vi "Init Controls.vi"(8 "error in":errorcluster, 10 "Disabled Controls":string[](array[string]), 11 "VI ref":refnum<vi>) -> (0 "error out":errorcluster)   [LabVIEW 2018]
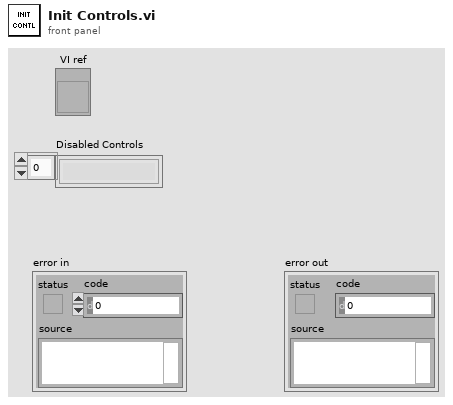
[diagram p1: front panel]
types:
  T1 = enum8{"Enabled", "Disabled", "Disabled and Grayed Out"}
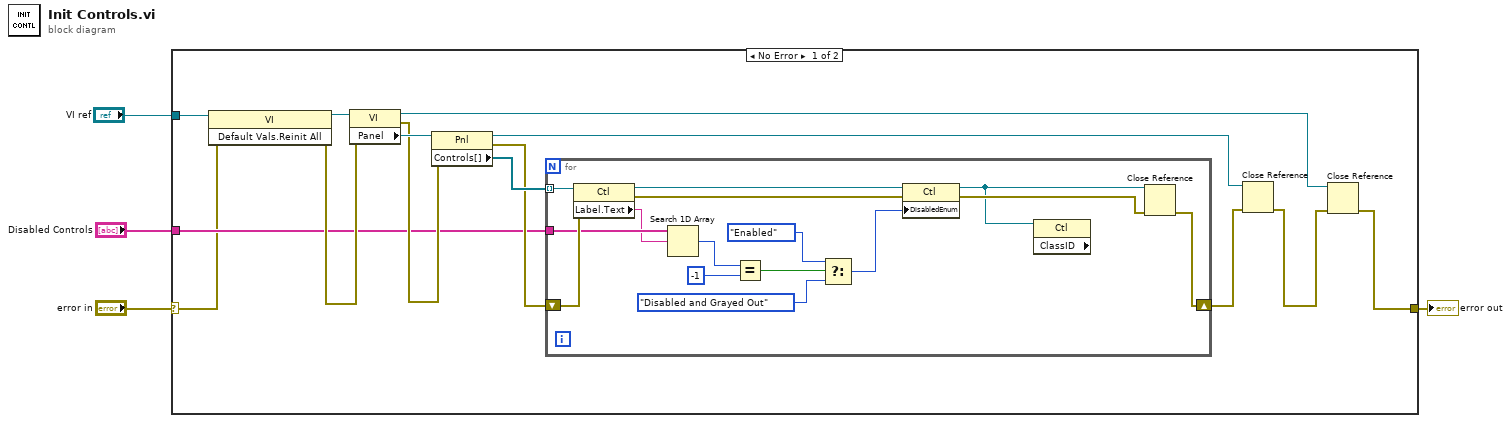
[diagram p0: block diagram]
diagram:
  n1 = case shown="No Error" "error in" {
    selector: "error in" -> [w10 w34]
    tunnel: "VI ref" -> [w18 _]
    tunnel: [w5 w34] -> w2
    tunnel: "Disabled Controls" -> [w11 _]
    frame No Error {
      n2 = invoke class="VI" method="Default Vals.Reinit All"(reference=w18, error in=w10) -> (reference out=w17:refnum<vi>, error out=w16:errorcluster)  [unwired: 1 in, 1 out]
      n3 = property class="VI"(reference=w17, error in=w16) -> (reference out=w6:refnum<vi>, error out=w14:errorcluster, "Panel"=w15:refnum<vi>)
      n4 = property class="Pnl"(reference=w15, error in=w14) -> (reference out=w9:refnum<vi>, error out=w12:errorcluster, "Controls[]"=w13:refnum<vi>[])
      n5 = for {
        shift-right: [w32] -> w8
        shift-left: w12 -> [w30]
        tunnel: w13 -> [w31] mode=indexing
        tunnel: w11 -> [w29]
        n6 = property class="Ctl"(reference=w31, error in=w30) -> (reference out=w27:refnum<vi>, error out=w26:errorcluster, "Label.Text"=w28:string)
        n7 = Search 1D Array(1D array=w29, element=w28) -> (index of element=w25:i32)  [unwired: 1 in]
        n8 = Equal?(x=w25, y=-1) -> (x = y?=w23:bool)
        n9 = Select(t=T1."Enabled" ("Disabled"), s=w23, f=T1."Disabled and Grayed Out" ("Disabled")) -> (s? t:f=w20:T1)
        n10 = property class="Ctl"(reference=w27, error in=w26, "DisabledEnum"=w20) -> (reference out=w19:refnum<vi>, error out=w33:errorcluster)
        n11 = property class="Ctl" props=["ClassID"](reference=w19) -> ()  [unwired: 1 in, 3 out]
        n12 = Close Reference(reference=w19, error in (no error)=w33) -> (error out=w32:errorcluster)
      }
      n13 = Close Reference(reference=w9, error in (no error)=w8) -> (error out=w7:errorcluster)
      n14 = Close Reference(reference=w6, error in (no error)=w7) -> (error out=w5:errorcluster)
    }
    frame Error {
    }
  }
  "error out" <- w2
